vi "dfd_Direct_FIR_T_C.vi"() -> ()   [LabVIEW 2017, in "NI_DigFilterTemp.lvlib"]
uses:
  <vilib>/addons/Digital Filter Design/NI_DigFilterTemp.lvlib
panel:
  in  "String":string="\n\n/* ---- Constants ----*/\n#define %CapName%_N_TAPS %kTAPS%\n#define %CapName%_N_STATES %CapName%_N_TAPS\n\n/* ---- Global Variables Declaration ----*/\nstatic %CoefBType% %FilterBlkName%_Coef[%CapName%_N_TAPS];\n%InternalFunctionsDeclaration%\n\n%ShiftDefine%\n\n%AssistantFunctions%\n\n/* ---- Implement the Fixed-Point Filter ---- */ \n%OutType% %FilterBlkName%_Filtering (%InType% sampleIn, %FilterBlkName%_State state)\n{\n\tI32 accA, accB;\n\t%InType% mult;\n\tint i;\n\n\tmult = (sampleIn << IN2MULT);\n\n\t/* Filtering */\n\taccA = accB = 0;\n\tfor (i = %CapName%_N_STATES-1; i >= 0 ; i--)\n\t{\n\t\taccA = accB + (%FilterBlkName%_%MultB%(mult, %FilterBlkName%_Coef[i]) << PROD2SUM);\n\t\taccB = (state[i] << DELAY2SUM);\n\t\tstate[i] = (accA << SUM2DELAY);\n\t}\n\n\t%ApplyGainAccA%\n\n\treturn (%OutType%)accA;\n}\n\n/* ---- Internal Functions ---- */\n%InternalFunctions%\n\n/* ---- Filter Coefficients ---- */\nstatic %CoefBType% %FilterBlkName%_Coef[] = {\n%CoefficientsB%\n};\n"
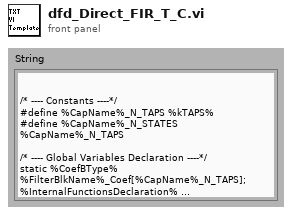
[diagram p1: front panel]
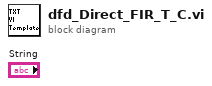
[diagram p0: block diagram]
diagram:
